vi "CSM - Run Script with Variable Support.vi"(0 "CSM Scripts":string, 1 "Current Module (\"\" to Generate an ID)":string, 7 "Continue If Error? (F)":bool, 9 "Wait (5000ms)":i32=5000, 11 "error in (no error)":errorcluster, 12 "Response Timeout (-2 Using Global Settings)":i32=-2) -> (4 "Response":string[](array[string]), 10 "Scripts Left":string, 15 "error out":errorcluster)   [LabVIEW 2020]
doc: "Executes multiple CSM commands in a single batch, supporting synchronous messages, asynchronous messages, and registrations.\n\n\n> [!NOTE] <b>CSM Message Target Module Description</b>\n>\n> In Normal Mode, the target module for a CSM message is the specified module name.\n> System-level modules start with a `.` in their name. The target module for a CSM message includes the `.` in the name. For example, if the requested module name is `.System`, the target module for the CSM message is `.System`.\n> In Worker Mode, the target module for a CSM message can only be the overall module name, not the node name. For example, if the requested module name is `Worker#`, the target module for the CSM message is `Worker`.\n> In Chain of Responsibility Mode, the target module for a CSM message can only be the overall module name, not the node name. For example, if the requested module name is `Chain$1`, the target module for the CSM message is `Chain`.\n\n\n-- <b>Controls</b> --\n- <b>Current Module (\"\" to Generate an ID)</b>: Name of the current module. If empty, a temporary ID is generated for debugging purposes to identify the location.\n- <b>CSM Scripts</b>: CSM commands to execute.\n- <b>Continue If Error? (F)</b>: Whether to continue execution if an error occurs. The default is FALSE, which specifies to not continue.\n- <b>Wait (5000 ms)</b>: Timeout duration for waiting module to be alive. The default is 5000 ms.\n- <b>Response Timeout (-2 Using Global Settings)</b>: Timeout for synchronous calls. The default is -2, which uses the global setting. You can set the global timeout using the CSM - Set TMO of Sync-Reply VI.\n\n-- <b>Indicators</b> --\n- <b>Response</b>: Returned results from executing the script. Only synchronous messages carry returns. The corresponding column for other commands will be an empty string.\n- <b>Scripts Left</b>: Remaining unexecuted scripts."
uses:
  <userlib>/_NEVSTOP/Communicable State Machine(CSM)/Communicable State Machine.lvlib
  <userlib>/_NEVSTOP/Communicable State Machine(CSM)/_Shared/CSM Shared.lvlib
  <userlib>/_NEVSTOP/Communicable State Machine(CSM)/AdvanceAPI/CSM - Broadcast Message Type.ctl
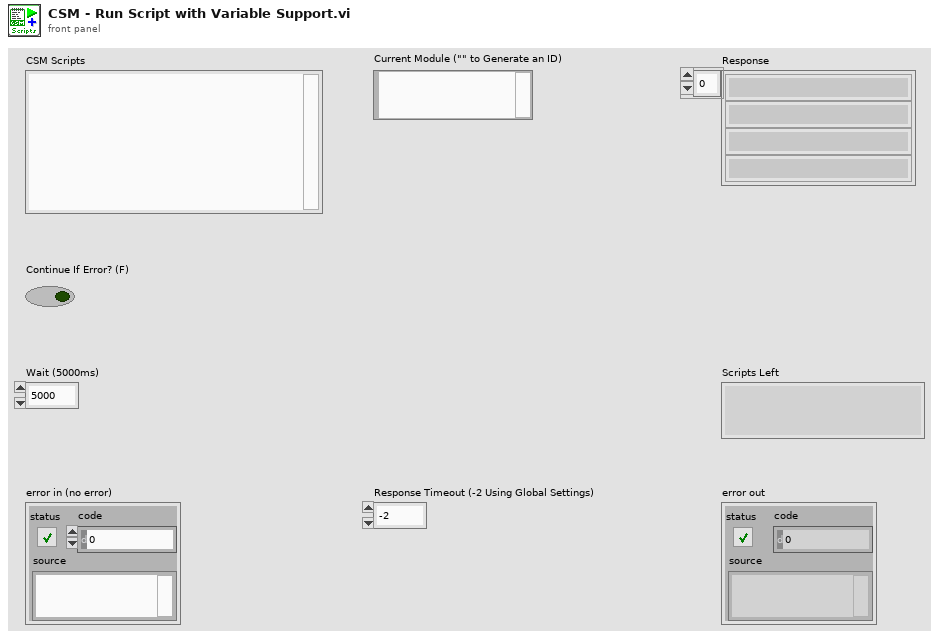
[diagram p1: front panel]
types:
  T1 = typedef "Communicable State Machine.lvlib/CSM - Broadcast Message Type.ctl" = enum16{"<Null>", "Status", "Interrupt"}
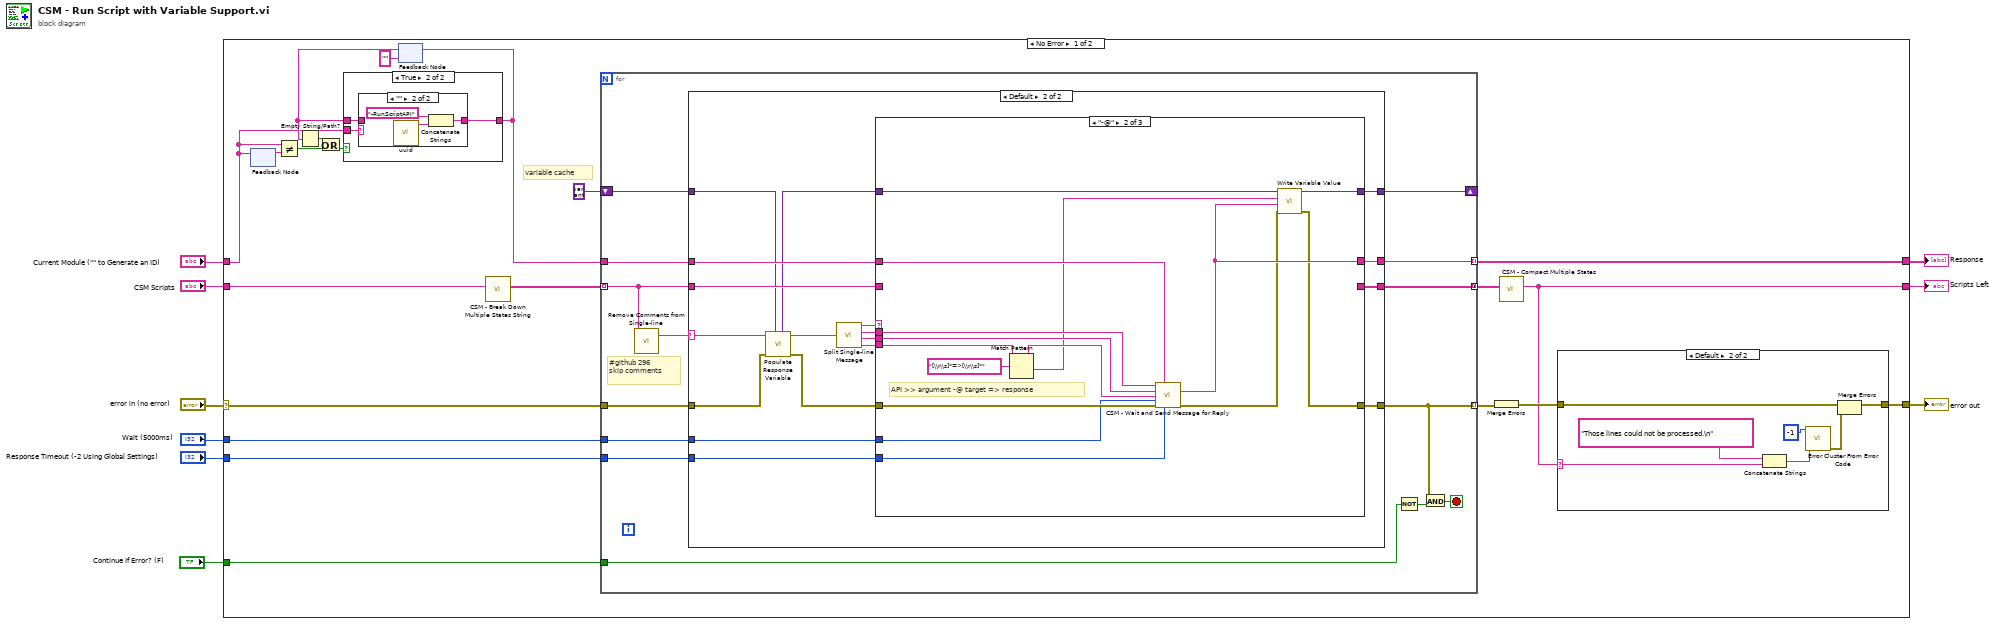
[diagram p0: block diagram]
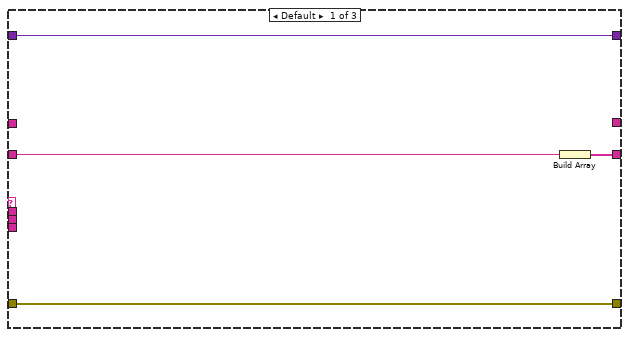
[diagram p6: hidden frame]
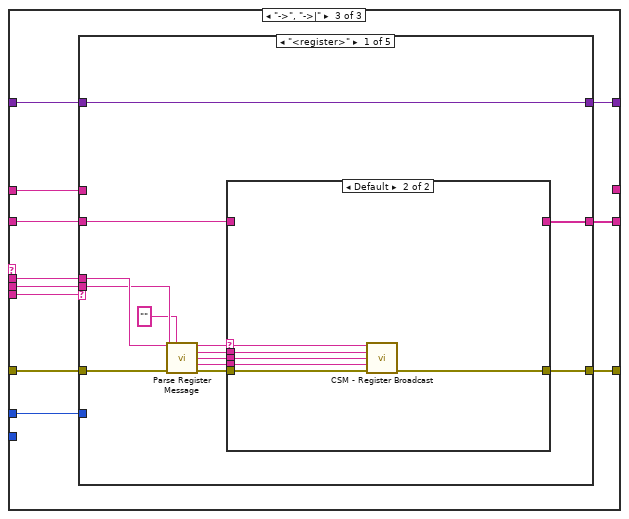
[diagram p7: hidden frame]
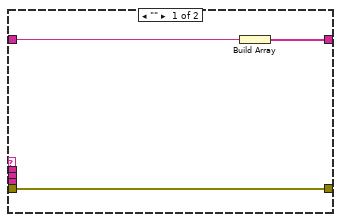
[diagram p8: hidden frame]
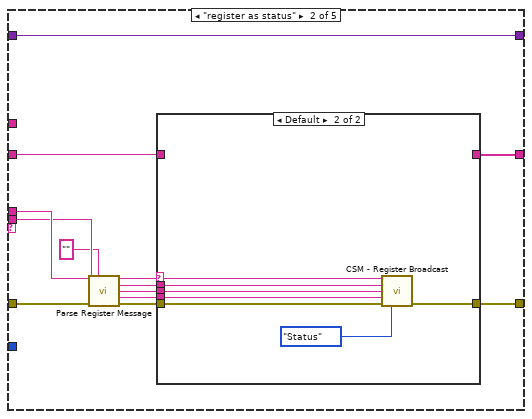
[diagram p9: hidden frame]
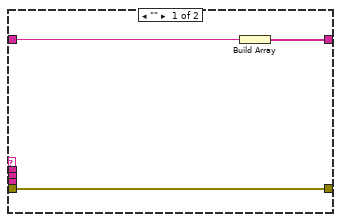
[diagram p10: hidden frame]
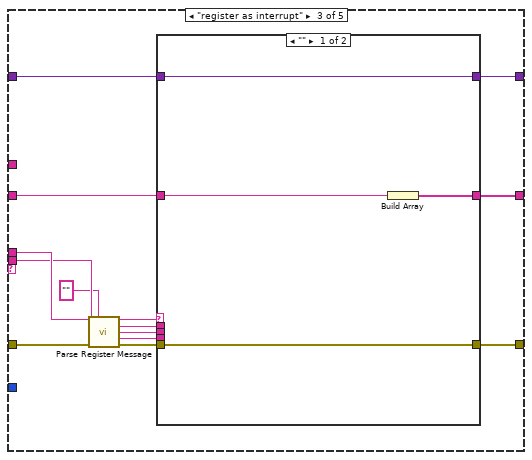
[diagram p11: hidden frame]
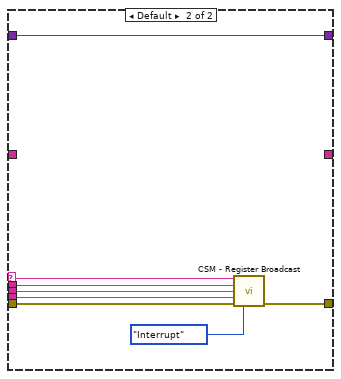
[diagram p12: hidden frame]
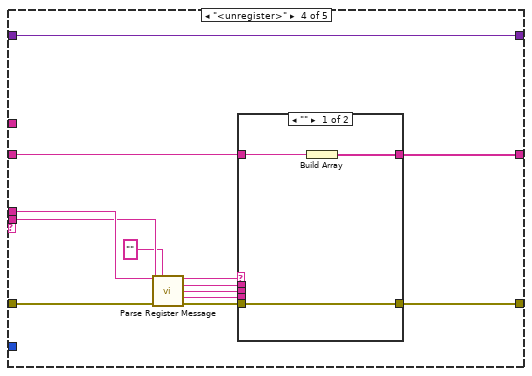
[diagram p13: hidden frame]
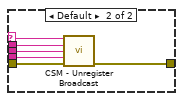
[diagram p14: hidden frame]
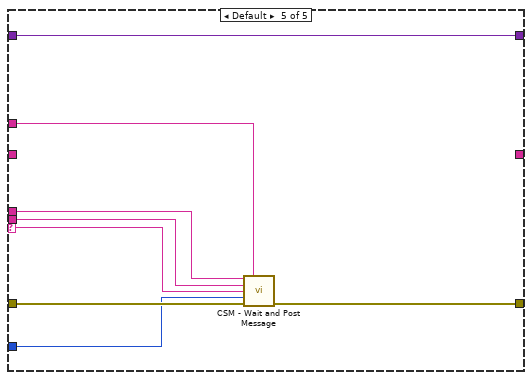
[diagram p15: hidden frame]
diagram:
  n1 = case shown="No Error" "error in (no error)" {
    selector: "error in (no error)" -> [w28 w208]
    tunnel: "CSM Scripts" -> [w27 _]
    tunnel: [w24 _] -> w7
    tunnel: [w23 w208] -> w6
    tunnel: "Current Module (\"\" to Generate an ID)" -> [w12 _]
    tunnel: "Response Timeout (-2 Using Global Settings)" -> [w22 _]
    tunnel: "Wait (5000ms)" -> [w21 _]
    tunnel: "Continue If Error? (F)" -> [w20 _]
    tunnel: [w19 _] -> w1
    frame No Error {
      # "variable cache"
      n2 = feedback #1() -> (w18:string)  [unwired: 1 in]
      n3 = feedback-in #1(w12) -> ()
      n4 = Not Equal?(x=w12, y=w18) -> (x != y?=w17:bool)
      n5 = feedback #2("") -> (w14:string)
      n6 = Empty String/Path?(string/path=w14) -> (empty?=w13:bool)
      n7 = Or(x=w13, y=w17) -> (x .or. y?=w15:bool)
      n8 = case shown="True" w15 {
        tunnel: w14 -> [w31 w34]
        tunnel: w12 -> [_ w33]
        tunnel: [w31 w32] -> w11
        frame False {
        }
        frame True {
          n9 = case shown="\"\"" w33 {
            selector: w33 -> [w35 _]
            tunnel: [w35 w36] -> w32
            tunnel: w34 -> [_ _]
            frame Default {
            }
            frame "" {
              n10 = call <userlib>:"uuid.vi"() -> ("UUID"=w37:string)  [unwired: 11 in]
              n11 = Concatenate Strings("-RunScriptAPI" ("Name (\"\" to Use UUID)"), w37) -> (w36:string)
            }
          }
        }
      }
      n12 = feedback-in #2(w11) -> ()
      n13 = call <userlib>:"CSM - Break Down Multiple States String.vi"("States"=w27) -> ("Multiple States"=w26:string[])  [unwired: 10 in]
      n14 = for {
        tunnel: w26 -> [w57] mode=indexing
        tunnel: w28 -> [w60]
        tunnel: [w52] -> w29 mode=indexing
        tunnel: [w58] -> w25 mode=concatenating
        tunnel: w11 -> [w56]
        tunnel: w22 -> [w55]
        tunnel: w21 -> [w54]
        tunnel: w20 -> [w51]
        tunnel: [w49] -> w19 mode=indexing
        shift-right: [w47] -> _
        shift-left: variant -> [w48]
        stop <- w53 stop-if-true
        # "#github 296\nskip comments"
        n15 = call <userlib>:"Remove Comments from Single-line.vi"("single-line text"=w57) -> ("single-line text without comments"=w59:string)  [unwired: 2 in]
        n16 = case shown="Default" w59 {
          selector: w59 -> [_ w66]
          tunnel: [w62 w80] -> w52
          tunnel: w60 -> [w62 w64]
          tunnel: [_ w75] -> w58
          tunnel: w57 -> [_ w74]
          tunnel: w56 -> [_ w73]
          tunnel: w55 -> [_ w72]
          tunnel: w54 -> [_ w71]
          tunnel: [_ w70] -> w49
          tunnel: w48 -> [w61 w68]
          tunnel: [w61 w69] -> w47
          frame "" {
          }
          frame Default {
            n17 = call "Populate Response Variable.vi"("Variant"=w68, "Error in"=w64, "String might with variables"=w66) -> ("Error out"=w63:errorcluster, "String out"=w65:string, "Variant Out"=w67:variant)  [unwired: 4 in]
            n18 = call <userlib>:"Split Single-line Message.vi"("single-line text"=w65) -> ("operator"=w79:string, "state"=w76:string, "args"=w77:string, "source/target"=w78:string)  [unwired: 6 in]
            n19 = case shown="\"-@\"" w79 {
              tunnel: w78 -> [_ w93 w110]
              tunnel: w77 -> [_ w99 w109]
              tunnel: w76 -> [_ w98 w108]
              tunnel: w63 -> [w84 w97 w107]
              tunnel: [w84 w85 w106] -> w80
              tunnel: [w83 _ w105] -> w75
              tunnel: w74 -> [w82 _ w104]
              tunnel: w73 -> [_ w96 w103]
              tunnel: w72 -> [_ w95 _]
              tunnel: w71 -> [_ w94 w102]
              tunnel: [_ w88 _] -> w70
              tunnel: [w81 w87 w101] -> w69
              tunnel: w67 -> [w81 w90 w100]
              frame Default {
                n20 = Build Array(w82) -> (w83:string[])
              }
              frame "-@" {
                # "API >> argument -@ target => response"
                n21 = Match Pattern(string=w93, regular expression="[\\r\\s]*=>[\\r\\s]*") -> (before substring=w91:string, after substring=w89:string)  [unwired: 1 in, 2 out]
                n22 = call <userlib>:"CSM - Wait and Send Message for Reply.vi"("State"=w98, "Current Module (\"\" to Generate an ID)"=w96, "Arguments (\"\")"=w99, "Target Module"=w91, "Wait (5000ms)"=w94, "Error In (No Error)"=w97, "Response Timeout (-2 Using Global Settings)"=w95) -> ("Response"=w88:string, "error out"=w86:errorcluster)  [unwired: 5 in, 2 out]
                n23 = call "Write Variable Value.vi"("Error in"=w86, "Response"=w88, "source/target"=w89, "Variant Out in"=w90) -> ("Error out"=w85:errorcluster, "Variant Out out"=w87:variant)  [unwired: 6 in]
              }
              frame "->", "->|" {
                n24 = case shown="\"<register>\"" w110 {
                  selector: w110 -> [_ _ _ _ w207]
                  tunnel: w109 -> [w117 w138 w161 w185 w206]
                  tunnel: w108 -> [w118 w139 w162 w186 w205]
                  tunnel: w107 -> [w116 w137 w160 w184 w204]
                  tunnel: [w115 w136 w159 w183 w203] -> w106
                  tunnel: [w113 w134 w157 w181 _] -> w105
                  tunnel: w104 -> [w112 w133 w156 w180 _]
                  tunnel: w103 -> [_ _ _ _ w202]
                  tunnel: w102 -> [_ _ _ _ w201]
                  tunnel: [w111 w132 w155 w179 w200] -> w101
                  tunnel: w100 -> [w111 w132 w154 w179 w200]
                  frame "<register>" {
                    n25 = call <userlib>:"Parse Register Message.vi"("State"=w118, "Module Name"="", "Args"=w117) -> ("Target"=w122:string, "Source"=w121:string, "Status"=w120:string, "Api"=w119:string)  [unwired: 8 in, 1 out]
                    n26 = case shown="Default" w122 {
                      selector: w122 -> [_ w131]
                      tunnel: w121 -> [_ w130]
                      tunnel: w120 -> [_ w129]
                      tunnel: w119 -> [_ w128]
                      tunnel: w116 -> [w125 w127]
                      tunnel: [w125 w126] -> w115
                      tunnel: [w123 _] -> w113
                      tunnel: w112 -> [w124 _]
                      frame "" {
                        n27 = Build Array(w124) -> (w123:string[])
                      }
                      frame Default {
                        n28 = call <userlib>:"CSM - Register Broadcast.vi"("CSM Name(Empty for Broadcast Event)"=w131, "Source CSM Name (* as Default)"=w130, "Trigger"=w129, "API (If \"\", Same as Trigger)"=w128, "Error In"=w127) -> ("error out"=w126:errorcluster)  [unwired: 9 in, 1 out]
                      }
                    }
                  }
                  frame "register as status" {
                    n29 = call <userlib>:"Parse Register Message.vi"("State"=w139, "Module Name"="", "Args"=w138) -> ("Target"=w143:string, "Source"=w142:string, "Status"=w141:string, "Api"=w140:string)  [unwired: 8 in, 1 out]
                    n30 = case shown="Default" w143 {
                      selector: w143 -> [_ w153]
                      tunnel: w142 -> [_ w152]
                      tunnel: w141 -> [_ w151]
                      tunnel: w140 -> [_ w150]
                      tunnel: w137 -> [w146 w149]
                      tunnel: [w146 w148] -> w136
                      tunnel: [w144 _] -> w134
                      tunnel: w133 -> [w145 _]
                      frame "" {
                        n31 = Build Array(w145) -> (w144:string[])
                      }
                      frame Default {
                        n32 = call <userlib>:"CSM - Register Broadcast.vi"("CSM Name(Empty for Broadcast Event)"=w153, "Source CSM Name (* as Default)"=w152, "Trigger"=w151, "API (If \"\", Same as Trigger)"=w150, "Error In"=w149, "Priority (No Change)"=CSM_-_Broadcast_Message_Type."Status") -> ("error out"=w148:errorcluster)  [unwired: 8 in, 1 out]
                      }
                    }
                  }
                  frame "register as interrupt" {
                    n33 = call <userlib>:"Parse Register Message.vi"("State"=w162, "Module Name"="", "Args"=w161) -> ("Target"=w166:string, "Source"=w165:string, "Status"=w164:string, "Api"=w163:string)  [unwired: 8 in, 1 out]
                    n34 = case shown="\"\"" w166 {
                      selector: w166 -> [_ w178]
                      tunnel: w165 -> [_ w177]
                      tunnel: w164 -> [_ w176]
                      tunnel: w163 -> [_ w175]
                      tunnel: w160 -> [w170 w174]
                      tunnel: [w170 w173] -> w159
                      tunnel: [w168 _] -> w157
                      tunnel: w156 -> [w169 _]
                      tunnel: [w167 w171] -> w155
                      tunnel: w154 -> [w167 w171]
                      frame "" {
                        n35 = Build Array(w169) -> (w168:string[])
                      }
                      frame Default {
                        n36 = call <userlib>:"CSM - Register Broadcast.vi"("CSM Name(Empty for Broadcast Event)"=w178, "Source CSM Name (* as Default)"=w177, "Trigger"=w176, "API (If \"\", Same as Trigger)"=w175, "Error In"=w174, "Priority (No Change)"=CSM_-_Broadcast_Message_Type."Interrupt") -> ("error out"=w173:errorcluster)  [unwired: 8 in, 1 out]
                      }
                    }
                  }
                  frame "<unregister>" {
                    n37 = call <userlib>:"Parse Register Message.vi"("State"=w186, "Module Name"="", "Args"=w185) -> ("Target"=w190:string, "Source"=w189:string, "Status"=w188:string, "Api"=w187:string)  [unwired: 8 in, 1 out]
                    n38 = case shown="\"\"" w190 {
                      selector: w190 -> [_ w199]
                      tunnel: w189 -> [_ w198]
                      tunnel: w188 -> [_ w197]
                      tunnel: w187 -> [_ w196]
                      tunnel: w184 -> [w193 w195]
                      tunnel: [w193 w194] -> w183
                      tunnel: [w191 _] -> w181
                      tunnel: w180 -> [w192 _]
                      frame "" {
                        n39 = Build Array(w192) -> (w191:string[])
                      }
                      frame Default {
                        n40 = call <userlib>:"CSM - Unregister Broadcast.vi"("CSM Name(Empty for Broadcast Event)"=w199, "Source CSM Name (* as Default)"=w198, "Trigger"=w197, "API (\"*\" as Default)"=w196, "Error In"=w195) -> ("error out"=w194:errorcluster)  [unwired: 9 in, 1 out]
                      }
                    }
                  }
                  frame Default {
                    n41 = call <userlib>:"CSM - Wait and Post Message.vi"("State"=w205, "Current Module (\"\" to Generate an ID)"=w202, "Arguments (\"\")"=w206, "Target Module"=w207, "Wait (5000ms)"=w201, "Error In (No Error)"=w204) -> ("error out"=w203:errorcluster)  [unwired: 8 in, 1 out]
                  }
                }
              }
            }
          }
        }
        n42 = Not(x=w51) -> (.not. x?=w50:bool)
        n43 = And(x=w52, y=w50) -> (x .and. y?=w53:bool)
      }
      n44 = Merge Errors(w29) -> (w30:errorcluster)
      n45 = call <userlib>:"CSM - Compact Multiple States.vi"("Multiple States"=w25) -> ("States"=w24:string)  [unwired: 9 in]
      n46 = case shown="Default" w24 {
        selector: w24 -> [_ w42]
        tunnel: w30 -> [w39 w46]
        tunnel: [w39 w41] -> w23
        frame "" {
        }
        frame Default {
          n47 = Concatenate Strings("Those lines could not be processed.\n" ("String to Prepend to source (\"\")"), w42) -> (w43:string)
          n48 = call <vilib>:"Error Cluster From Error Code.vi"("error message (\"\")"=w43, "error code (0)"=-1 ("code")) -> ("error out"=w40:errorcluster)  [unwired: 7 in]
          n49 = Merge Errors(w46, w40) -> (w41:errorcluster)
        }
      }
    }
    frame Error {
    }
  }
  "error out" <- w6
  "Scripts Left" <- w7
  "Response" <- w1
